vi "ALTS-2015 Decide Next Task.vi"(8 "error in (no error)":errorcluster, 11 "Task Details":T1[](array[typedef])) -> (0 "error out":errorcluster, 3 "Remaining Tasks":T1[](array[typedef]), 5 "Found?":bool, 7 "Next Task to Perform":T1)   [LabVIEW 2013]
uses:
  Controls/ALTS-2015 Serial Details.ctl
  Controls/ALTS-2015 Robot Tasks.ctl
  Controls/ALTS-2015 Station Cluster.ctl
  Controls/ALTS-2015 Serial DB Details.ctl
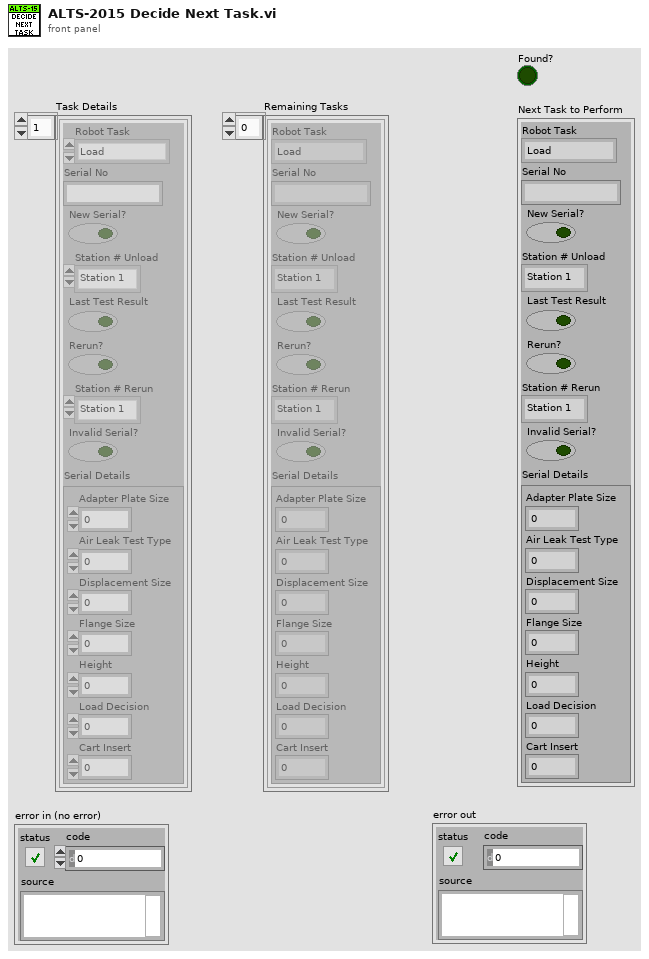
[diagram p1: front panel]
types:
  T1 = typedef "ALTS-2015 Serial Details.ctl" = cluster{"Robot Task":T2, "Serial No":string, "New Serial?":bool, "Station # Unload":T3, "Last Test Result":bool, "Rerun?":bool, "Station # Rerun":T3, "Invalid Serial?":bool, "Serial Details":T4}
  T2 = typedef "ALTS-2015 Robot Tasks.ctl" = enum16{"Load", "Unload", "Rerun", "Invalid Serial"}
  T3 = typedef "ALTS-2015 Station Cluster.ctl" = enum16{"Station 1", "Station 2", "Station 3", "Station 4"}
  T4 = typedef "ALTS-2015 Serial DB Details.ctl" = cluster{"Adapter Plate Size":i32, "Air Leak Test Type ":i32, "Displacement Size":i32, "Flange Size":i32, "Height":i32, "Load Decision":i32, "Cart Insert":i32}
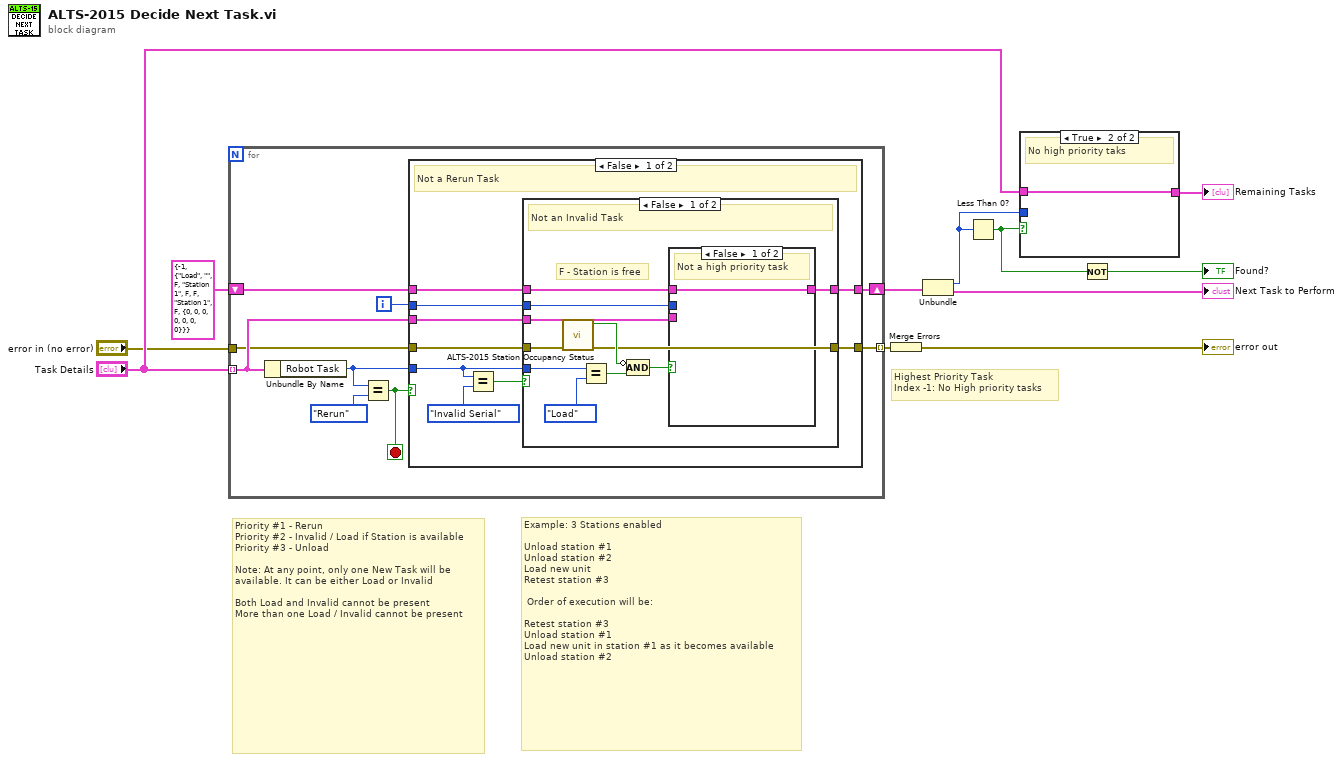
[diagram p0: block diagram]
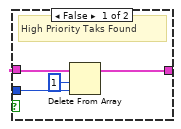
[diagram p2: hidden frame]
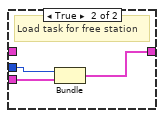
[diagram p3: hidden frame]
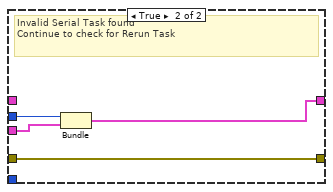
[diagram p4: hidden frame]
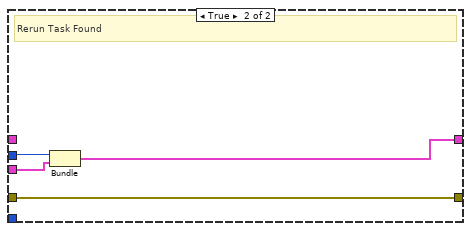
[diagram p5: hidden frame]
diagram:
  # "Highest Priority Task\nIndex -1: No High priority tasks"
  # "Example: 3 Stations enabled\n\nUnload station #1\nUnload station #2\nLoad new unit\nRetest station #3\n\n Order of execution will be:\n\nRetest station #3\nUnload station #1\nLoad new unit in station #1 as it becomes available\nUnload station #2"
  # "Priority #1 - Rerun\nPriority #2 - Invalid / Load if Station is available\nPriority #3 - Unload\n\nNote: At any point, only one New Task will be available. It can be either Load or Invalid\n\nBoth Load and Invalid cannot be present\nMore than one Load / Invalid cannot be present"
  n1 = for {
    tunnel: "Task Details" -> [w19] mode=indexing
    shift-right: [w17] -> w7
    shift-left: cluster{"Index":i32, "Part Details":T1} {"Index"=-1, "Part Details"={"Robot Task"=enum."Load", "Serial No"="", "New Serial?"=FALSE, "Station # Unload"=enum."Station 1", "Last Test Result"=FALSE, "Rerun?"=FALSE, "Station # Rerun"=enum."Station 1", "Invalid Serial?"=FALSE, "Serial Details"={"Adapter Plate Size"=0, "Air Leak Test Type "=0, "Displacement Size"=0, "Flange Size"=0, "Height"=0, "Load Decision"=0, "Cart Insert"=0}}} -> [w14]
    tunnel: "error in (no error)" -> [w13]
    tunnel: [w12] -> w4 mode=indexing
    i -> [w18]
    stop <- w15 stop-if-true
    n2 = Unbundle By Name(w19) -> ("Robot Task"=w16:T2)
    n3 = Equal?(x=w16, y=ALTS-2015_Robot_Tasks."Rerun") -> (x = y?=w15:bool)
    n4 = case shown="False" w15 {
      tunnel: w19 -> [w26 w51]
      tunnel: w18 -> [w27 w52]
      tunnel: [w25 w50] -> w17
      tunnel: w16 -> [w24 _]
      tunnel: w14 -> [w23 _]
      tunnel: w13 -> [w22 w49]
      tunnel: [w21 w49] -> w12
      frame False {
        # "Not a Rerun Task"
        n5 = Equal?(x=w24, y=ALTS-2015_Robot_Tasks."Invalid Serial") -> (x = y?=w28:bool)
        n6 = case shown="False" w28 {
          tunnel: w27 -> [w35 w48]
          tunnel: w26 -> [w34 w47]
          tunnel: [w33 w46] -> w25
          tunnel: w24 -> [w39 _]
          tunnel: w23 -> [w32 _]
          tunnel: w22 -> [w31 w45]
          tunnel: [w30 w45] -> w21
          frame False {
            # "F - Station is free"
            # "Not an Invalid Task"
            n7 = call "ALTS-2015 Station Occupancy Status.vi"("error in"=w31) -> ("error out"=w30:errorcluster, "Station Unavailable"=w38:bool)  [unwired: 8 in, 1 out]
            n8 = Equal?(x=w39, y=ALTS-2015_Robot_Tasks."Load") -> (x = y?=w37:bool)
            n9 = Compound Arithmetic op=AND(invert w38, w37) -> (w36:bool)
            n10 = case shown="False" w36 {
              tunnel: w35 -> [_ w44]
              tunnel: w34 -> [_ w43]
              tunnel: [w41 w42] -> w33
              tunnel: w32 -> [w41 _]
              frame False {
                # "Not a high priority task"
              }
              frame True {
                # "Load task for free station"
                n11 = Bundle(w44, "Part Details"=w43) -> (w42:cluster{i32, "Part Details":T1})  [unwired: 1 in]
              }
            }
          }
          frame True {
            # "Invalid Serial Task found\nContinue to check for Rerun Task"
            n12 = Bundle(w48, "Part Details"=w47) -> (w46:cluster{i32, "Part Details":T1})  [unwired: 1 in]
          }
        }
      }
      frame True {
        # "Rerun Task Found"
        n13 = Bundle(w52, "Part Details"=w51) -> (w50:cluster{i32, "Part Details":T1})  [unwired: 1 in]
      }
    }
  }
  n14 = Merge Errors(w4) -> (→"error out":errorcluster)
  n15 = Unbundle(w7) -> ("Index"=w9:i32, "Part Details"=→"Next Task to Perform":T1)
  n16 = Less Than 0?(x=w9) -> (x < 0?=w8:bool)
  n17 = case shown="True" w8 {
    tunnel: w9 -> [w55 _]
    tunnel: "Task Details" -> [w54 w57]
    tunnel: [w53 w57] -> w1
    frame False {
      # "High Priority Taks Found"
      n18 = Delete From Array(array=w54, length=1, index=w55) -> (array with subset deleted=w53:T1[])  [unwired: 1 out]
    }
    frame True {
      # "No high priority taks"
    }
  }
  "Remaining Tasks" <- w1
  n19 = Not(x=w8) -> (.not. x?=→"Found?":bool)
